vi "PROXY_prepare_diagnostics_record_for_buffer.vi"(5 "station":T1, 7 "message_type":T3, 8 "to":string, 9 "from":string, 10 "message":string, 11 "station_name":string) -> (3 "record":T2)   [LabVIEW 2020]
uses:
  _misc/DIAGNOSTICS_message_type.ctl
  FGV/DIAGNOSTICS_message_history_buffer/PROXY_DIAGNOSTICS_message_history_buffer_all_info.ctl
  STATION/station.ctl
  _misc/AULocalize/SubVIs/Get Localized Phrase Compact Interface 0D.vi
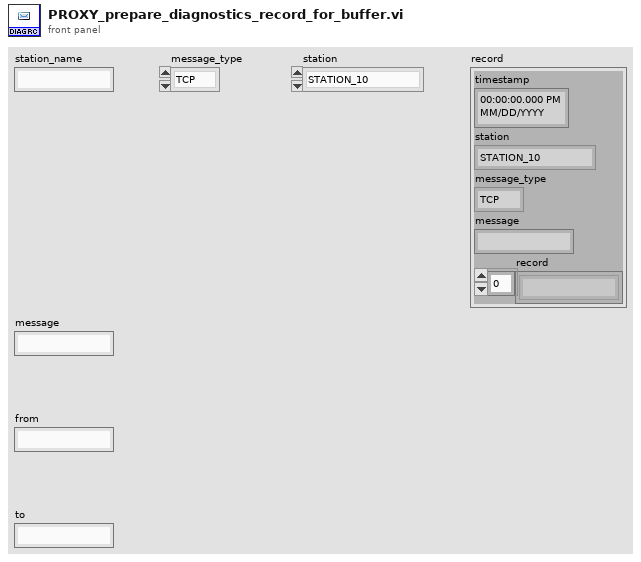
[diagram p1: front panel]
types:
  T1 = typedef "station.ctl" = enum16{"STATION_10", "STATION_20", "STATION_30", "STATION_40", "STATION_50", "STATION_60", "STATION_70", "STATION_80", "STATION_90", "STATION_100", "STATION_110", "STATION_120", "STATION_165", "MAIN"}
  T2 = typedef "PROXY_DIAGNOSTICS_message_history_buffer_all_info.ctl" = cluster{"timestamp":timestamp, "station":T1, "message_type":T3, "message":string, "record":string[]}
  T3 = typedef "DIAGNOSTICS_message_type.ctl" = enum16{"TCP", "SQL"}
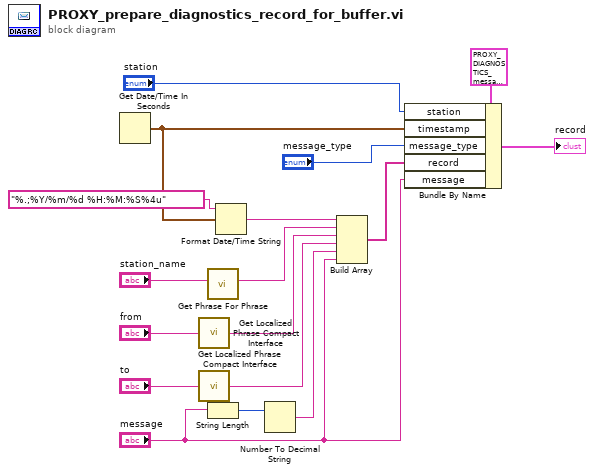
[diagram p0: block diagram]
diagram:
  n1 = Get Date/Time In Seconds() -> (seconds since 1Jan1904=w8:timestamp)
  n2 = call-poly "Get Localized Phrase Compact Interface.vi"("Key"="from") -> ("Translated Phrase"=w4:string)
  n3 = call-poly "Get Localized Phrase Compact Interface.vi"("Key"="to") -> ("Translated Phrase"=w3:string)
  n4 = call "Get Phrase For Phrase.vi"("Phrase"="station_name") -> ("Phrase"=w1:string)  [unwired: 9 in, 1 out]
  n5 = String Length(string="message") -> (length=w7:i32)
  n6 = Format Date/Time String(time format string (%c)="%.;%Y/%m/%d %H:%M:%S%4u", seconds (now)=w8) -> (date/time string=w14:string)  [unwired: 1 in]
  n7 = Number To Decimal String(number=w7) -> (decimal integer string=w6:string)  [unwired: 1 in]
  n8 = Build Array(w14, w1, w4, w3, w6, "message") -> (w15:string[])
  n9 = Bundle By Name(cluster=T2 {"timestamp"=timestamp(0 s since 1904-01-01), "station"=enum."STATION_10", "message_type"=enum."TCP", "message"="", "record"=[]} ("Cluster"), "station"="station", "timestamp"=w8, "message_type"="message_type", "record"=w15, "message"="message") -> (→"record":T2)
